vi "AIM 664 test Add Multiple Custom Devices.vi"(8 "error in (no error)":errorcluster, 11 "TestCase in":refnum<class "AIM 664 Scripting.lvclass">) -> (0 "error out":errorcluster, 3 "TestCase out":refnum<class "AIM 664 Scripting.lvclass">)   [LabVIEW 2020, in "AIM 664 Scripting.lvclass"]
uses:
  AIM 664 Scripting.lvclass
  C:/Program Files (x86)/National Instruments/LabVIEW 2020/vi.lib/NI/VeriStand Custom Device Testing Tools/VeriStandScriptingTestCase/VeriStandScriptingTestCase.lvclass
  <vilib>/NI/VeriStand Custom Device Testing Tools/VeriStandScriptingTestCase/VeriStandScriptingTestCase.lvclass/VeriStandScriptingTestCase.ctl
  <vilib>/NI/VeriStand Custom Device Testing Tools/VeriStandScriptingTestCase/Read Target.vi
  NationalInstruments.VeriStand.SystemDefinitionAPI
  <vilib>/addons/_JKI Toolkits/VI Tester/TestCase.llb/TestCase.lvclass
  Scripting/AIM ARINC 664 Scripting.lvlib
  C:/Program Files (x86)/National Instruments/LabVIEW 2020/vi.lib/addons/_JKI Toolkits/VI Tester/TestCase.llb/TestCase.lvclass
  C:/repos/niveristand-aim-arinc664-custom-device/Source/Custom Device Support/Tests/Unit/Scripting/AIM 664 Scripting.lvclass
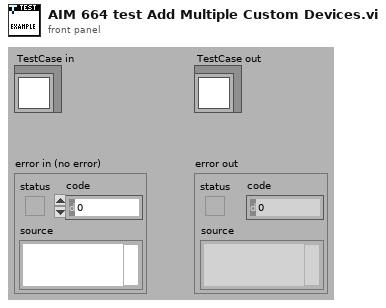
[diagram p1: front panel]
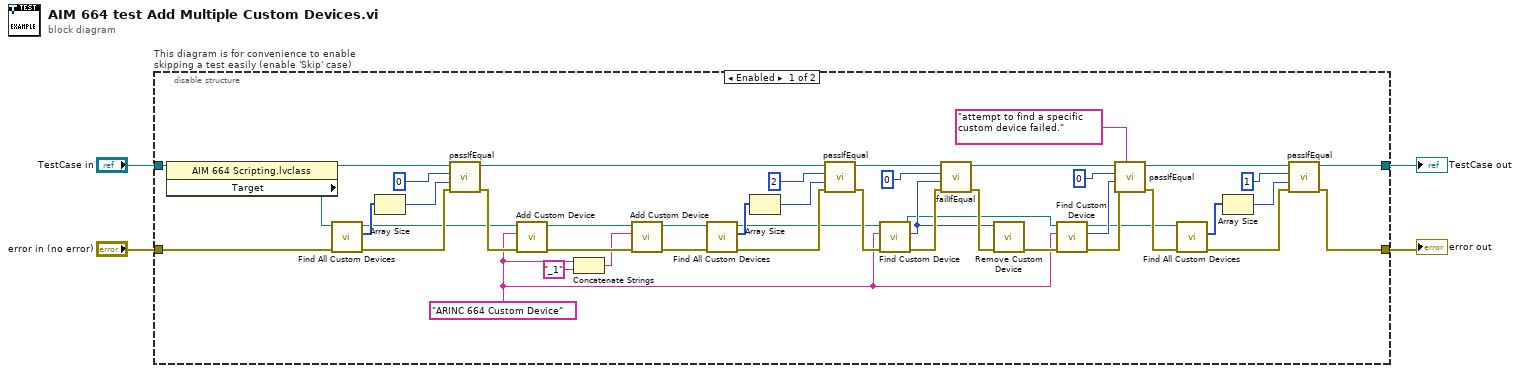
[diagram p0: block diagram]
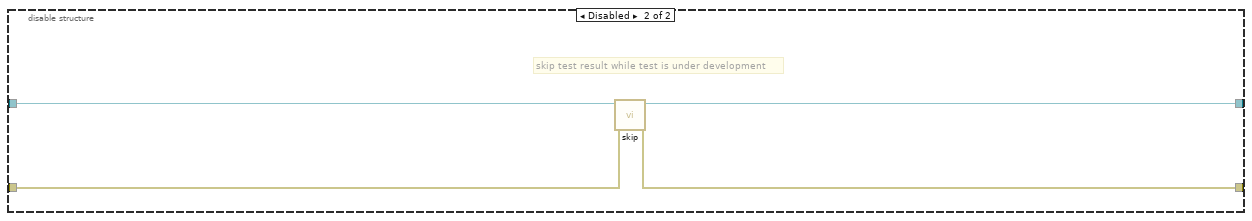
[diagram p2: hidden frame]
diagram:
  n1 = disable-structure "This diagram is for convenience to enable skipping a test easily (enable 'Skip' case)" shown="Enabled" {
    disable-tunnel: "TestCase in" -> [w6 w53]
    disable-tunnel: [w7 w51] -> w1
    disable-tunnel: [w8 w52] -> w3
    disable-tunnel: "error in (no error)" -> [w9 w50]
    frame Enabled {
      w25 = "ARINC 664 Custom Device" ("name")
      n2 = property class="AIM 664 Scripting.lvclass"(reference=w6) -> (reference out=w10:refnum<class "AIM 664 Scripting.lvclass">, "Target"=w11:refnum<k24>)  [unwired: 1 in, 1 out]
      n3 = call "Find All Custom Devices.vi"("error in"=w9, "target in"=w11) -> ("error out"=w46:errorcluster, "custom devices"=w49:u64[], "target out"=w44:refnum<k24>)  [unwired: 7 in]
      n4 = Array Size(array=w49) -> (size(s)=w48:i32)
      n5 = call-dynamic "passIfEqual.vi"("error in (no error)"=w46, "y"=w48, "x"=0 ("size(s)"), "TestCase in"=w10) -> ("error out"=w45:errorcluster, "TestCase out"=w34:refnum<class "AIM 664 Scripting.lvclass">)  [unwired: 6 in]
      n6 = call "Add Custom Device.vi"("error in"=w45, "name"=w25, "target in"=w44) -> ("error out"=w42:errorcluster, "target out"=w41:refnum<k24>)  [unwired: 6 in, 1 out]
      n7 = Concatenate Strings(w25, "_1" ("string")) -> (w40:string)
      n8 = call "Add Custom Device.vi"("error in"=w42, "name"=w40, "target in"=w41) -> ("error out"=w39:errorcluster, "target out"=w38:refnum<k24>)  [unwired: 6 in, 1 out]
      n9 = call "Find All Custom Devices.vi"("error in"=w39, "target in"=w38) -> ("error out"=w33:errorcluster, "custom devices"=w35:u64[], "target out"=w31:refnum<k24>)  [unwired: 7 in]
      n10 = Array Size(array=w35) -> (size(s)=w36:i32)
      n11 = call-dynamic "passIfEqual.vi"("error in (no error)"=w33, "y"=w36, "x"=2 ("size(s)"), "TestCase in"=w34) -> ("error out"=w32:errorcluster, "TestCase out"=w30:refnum<class "AIM 664 Scripting.lvclass">)  [unwired: 6 in]
      n12 = call "Find Custom Device.vi"("error in"=w32, "name"=w25, "target in"=w31) -> ("error out"=w29:errorcluster, "custom device"=w27:u64, "target out"=w24:refnum<k24>)  [unwired: 6 in]
      n13 = call-dynamic "failIfEqual.vi"("error in (no error)"=w29, "y"=w27, "x"=u64 0 ("custom device"), "TestCase in"=w30) -> ("error out"=w28:errorcluster, "TestCase out"=w23:refnum<class "AIM 664 Scripting.lvclass">)  [unwired: 6 in]
      n14 = call "Remove Custom Device.vi"("error in"=w28, "custom device"=w27) -> ("error out"=w26:errorcluster)  [unwired: 9 in]
      n15 = call "Find Custom Device.vi"("error in"=w26, "name"=w25, "target in"=w24) -> ("error out"=w19:errorcluster, "custom device"=w21:u64, "target out"=w17:refnum<k24>)  [unwired: 6 in]
      n16 = call-dynamic "passIfEqual.vi"("custom report message (\"\")"="attempt to find a specific custom device failed." ("message (\"\")"), "error in (no error)"=w19, "y"=w21, "x"=u64 0 ("custom device"), "TestCase in"=w23) -> ("error out"=w18:errorcluster, "TestCase out"=w15:refnum<class "AIM 664 Scripting.lvclass">)  [unwired: 5 in]
      n17 = call "Find All Custom Devices.vi"("error in"=w18, "target in"=w17) -> ("error out"=w14:errorcluster, "custom devices"=w13:u64[])  [unwired: 7 in, 1 out]
      n18 = Array Size(array=w13) -> (size(s)=w12:i32)
      n19 = call-dynamic "passIfEqual.vi"("error in (no error)"=w14, "y"=w12, "x"=1 ("size(s)"), "TestCase in"=w15) -> ("error out"=w8:errorcluster, "TestCase out"=w7:refnum<class "AIM 664 Scripting.lvclass">)  [unwired: 6 in]
    }
    frame Disabled {
      # "skip test result while test is under development"
      n20 = call <vilib>:"skip.vi"("error in (no error)"=w50, "TestCase in"=w53) -> ("error out"=w52:errorcluster, "TestCase out"=w51:refnum<class "AIM 664 Scripting.lvclass">)  [unwired: 8 in]
    }
  }
  "error out" <- w3
  "TestCase out" <- w1
